vi "Update Config.vi"(8 "error in (no error)":errorcluster, 11 "Config Updater in":refnum<class "Config Updater.lvclass">) -> (0 "error out":errorcluster)   [LabVIEW 2020, in "Volatus.lvlib" / "Config Updater.lvclass"]
uses:
  Config Updater.lvclass
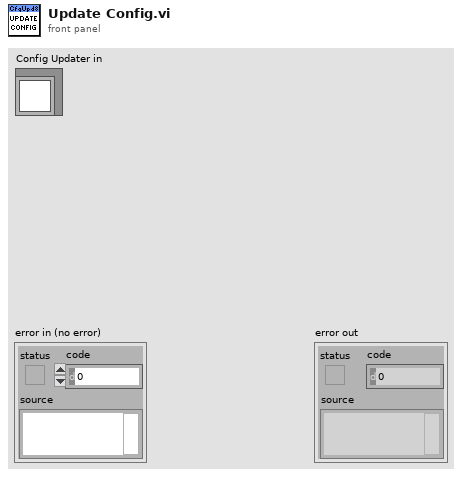
[diagram p1: front panel]
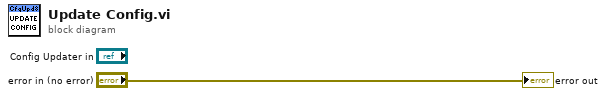
[diagram p0: block diagram]
diagram:
  "error out" <- "error in (no error)"
